vi "Intake Handler.vi"(11 "JoystickDevRef":T1) -> ()   [LabVIEW 2019]
uses:
  <vilib>/Rock Robotics/WPI/Joystick/WPI_JoystickDevRef.ctl
  <vilib>/Rock Robotics/WPI/Joystick/WPI_JoystickDeviceEnum.ctl
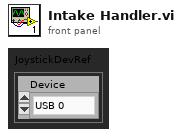
[diagram p1: front panel]
types:
  T1 = typedef "WPI_JoystickDevRef.ctl" = cluster{"Device":T2}
  T2 = typedef "WPI_JoystickDeviceEnum.ctl" = enum16{"USB 0", "USB 1", "USB 2", "USB 3", "USB 4", "USB 5"}
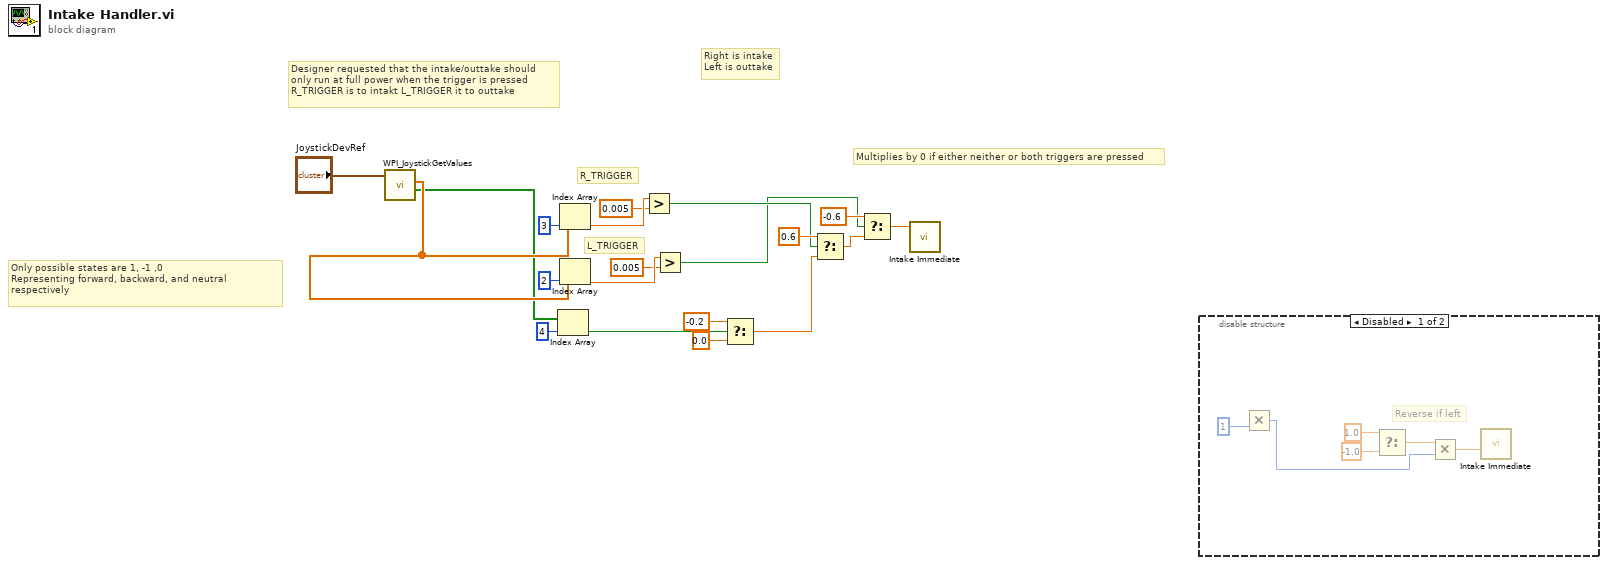
[diagram p0: block diagram]
diagram:
  # "Right is intake\nLeft is outtake"
  # "Multiplies by 0 if either neither or both triggers are pressed"
  # "R_TRIGGER"
  # "L_TRIGGER"
  # "Only possible states are 1, -1 ,0\nRepresenting forward, backward, and neutral respectively"
  # "Designer requested that the intake/outtake should \nonly run at full power when the trigger is pressed\nR_TRIGGER is to intakt L_TRIGGER it to outtake"
  n1 = call <vilib>:"WPI_JoystickGetValues.vi"("JoystickDevRef"="JoystickDevRef") -> ("Buttons"=w6:bool[], "Axes"=w19:dbl[])  [unwired: 6 in, 3 out]
  n2 = Index Array(array=w6, index=4) -> (element=w5:bool)
  n3 = Index Array(array=w19, index=3) -> (element=w18:dbl)
  n4 = Index Array(array=w19, index=2) -> (element=w17:dbl)
  n5 = Greater?(x=w18, y=0.005) -> (0:w9:bool)
  n6 = Greater?(x=w17, y=0.005) -> (0:w8:bool)
  n7 = Select(t=-0.2, s=w5, f=0.0) -> (s? t:f=w4:dbl)
  n8 = Select(t=0.6, s=w9, f=w4) -> (s? t:f=w11:dbl)
  n9 = Select(t=-0.6, s=w8, f=w11) -> (s? t:f=w1:dbl)
  n10 = call "Intake Immediate.vi"("Setpoint"=w1) -> ()  [unwired: 10 in, 1 out]
  n11 = disable-structure shown="Disabled" {
    frame Disabled {
      # "Reverse if left"
      n12 = Multiply(y=1) -> (x*y=w25:i32)  [unwired: 1 in]
      n13 = Select(t=1.0, f=-1.0) -> (s? t:f=w24:dbl)  [unwired: 1 in]
      n14 = Multiply(x=w24, y=w25) -> (x*y=w26:dbl)
      n15 = call "Intake Immediate.vi"("Setpoint"=w26) -> ()  [unwired: 10 in, 1 out]
    }
    frame Enabled {
    }
  }
